vi "Real time state machine - Saccade suppression.vi"() -> ()   [LabVIEW 2013]
uses:
  <vilib>/Platform/TimedLoop/XDataNode/timing_clust.ctl
  <vilib>/Platform/TimedLoop/XDataNode/nitl_modes.ctl
  <vilib>/Platform/TimedLoop/XDataNode/wakeup.ctl
  <vilib>/DAQmx/write.llb/DAQmx Write (Digital 1D Bool NChan 1Samp 1Line).vi
  <vilib>/DAQmx/read.llb/DAQmx Read (Analog 1D DBL NChan 1Samp).vi
  <vilib>/platform/TimedLoop/XDataNode/XDataNode.xnode
  <vilib>/Platform/TimedLoop/XDataNode/XDNodeRunTimeDep.lvlib
panel:
  out "Min":dbl
  out "Sec":dbl=47.16078567504883
  in  "Display length (S)":sgl=10.0
  out "shaft encoder":waveform(sgl)(graph)={"t0"=timestamp(3524542772.3366966 s since 1904-01-01), "dt"=0.02, "Y"=array[500 elements]}
  out "Current state":T1(ring)=enum."VS"
  out "# of rewards":i32
  in  "Automatic reward":bool=TRUE
  out "Lick reward":bool
  out "RT FIFO (DISP)":u32(slide) scale=0.0..50.0
  out "RT FIFO (Log)":u32(slide) scale=0.0..50.0
  out "Digital Waveform Graph":digitalwaveform(graph)={"t0"=timestamp(3524542772.3366966 s since 1904-01-01), "dt"=0.0004, "Y"={"transitions"=[], "data"=array25000x3[75000 elements]}, "error"={"status"=FALSE, "code"=37421928, "source"=""}}
  out "Trial # (State machine)":u32=1
  out "Actual cycle period (uS)":i64=94
  in  "State machine cycle (uS)":i64=200
  in  "Save file to":string="C:\\ni-rt\\LabVIEW Data\\"
  in  "RT FIFO size":u32=50
  in  "VS filter period (uS)":i32=500
  out "Start one trial":bool
  out "Trial Done":bool
  out "error out":errorcluster
  out "Busy":bool
  out "Trial #":i32=1
  out "Save data":bool
  out "LED?":bool
  out "Pulse amp 0":sgl
  out "Pulse amp 1":sgl
  out "Pulse delay":sgl
  out "Pulse width":sgl
  out "Pulse period (ms)":sgl
  out "Pulse #":sgl
  out "Reward period (uS)":u32
  out "Reward start delay (uS)":u32
  out "Water duration (uS)":u32=30000
  out "Water refractory period (uS)":u32=500000
  out "Shock duration (uS)":u32=10000
  out "Shock refractory period (uS)":u32=1000000
  out "Trial timeout (uS)":u32=3000000
  out "Lick threshold (V)":fxp<+,32,16>=1.600006103515625
  out "Track eye":bool=TRUE
  out "Allow shock":bool
  out "Allow timeout":bool
  out "Manually give water":bool
  out "Manually give shock":bool
  out "VS threshold (V)":fxp<+,32,16>=0.5
  out "VS type":string="continuous_flash"
  out "File name":string="Test"
  out "Behavior type":string="fullfield"
  in  "Stop state":bool
  in  "Remote port":u16=9090
  in  "Remote IP_Main":string="192.168.137.10"
  in  "Local port":u16=9091
  in  "Local IP_This computer":string="192.168.137.2"
  out "ABORT":bool
  out "Initial data received":bool
  # "VS"
  # "Behavior"
  # "Trial #"
  # "Received parameters"
  # "Time to wait for reward window"
  # "Elapsed time"
  # "Min"
  # "Sec"
  # "Controls"
  # "Network"
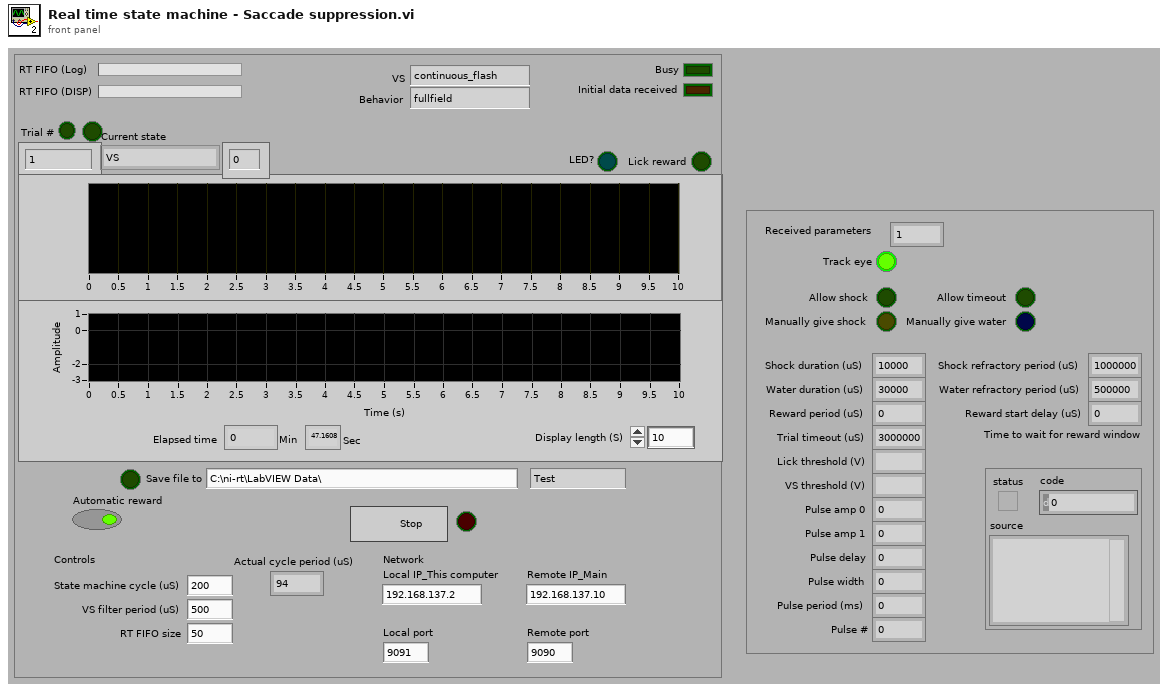
[diagram p1: front panel]
types:
  T1 = enum16{"Idle", "Before VS", "VS", "VS2", "After VS", "Wait for lever press", "Cycle End", "Reward", "Reward Refractory", "Punish", "Punish Refractory", "Exit", "Timeout", "Lick reward"}
  T2 = enum16{"open", "replace", "create", "open or create", "replace or create", "replace or create with confirmation"}
  T3 = typedef "XDNodeRunTimeDep.lvlib/timing_clust.ctl" = cluster{"Expected End [f-1]":u64, "Actual End [f-1]":u64, "Finished Late? [f-1]":bool, "Expected End [i-1]":u64, "Actual End [i-1]":u64, "Finished Late? [i-1]":bool, "Expected Start [i]":u64, "Actual Start [i]":u64, "Expected Start [f]":u64, "Actual Start [f]":u64, "Source Name":string, "Structure Name":string, "Period":i64, "Deadline":i64, "Offset":i64, "Start":i64, "Priority":i32, "Timeout":i32, "Mode":T4, "Wakeup Reason":T5, "Error":errorcluster, "Source Type":string, "Secondary Source Type":string, "Global End Time":u64, "Global Start Time":u64, "Frame Duration":u64, "Iteration Duration":u64, "Assigned CPU":i32, "I/O Scan Engine Mode":u32}
  T4 = typedef "XDNodeRunTimeDep.lvlib/nitl_modes.ctl" = enum32{"No Change", "Process missed periods, maintain original phase", "Discard missed periods, maintain original phase", "Process missed periods, ignore original phase", "Discard missed periods, ignore original phase"}
  T5 = typedef "XDNodeRunTimeDep.lvlib/wakeup.ctl" = enum32{"Normal", "Aborted", "Asynchronous wakeup", "Timing source error", "Timed loop error", "Timeout"}
  T6 = enum16{"big-endian, network order", "native, host order", "little-endian"}
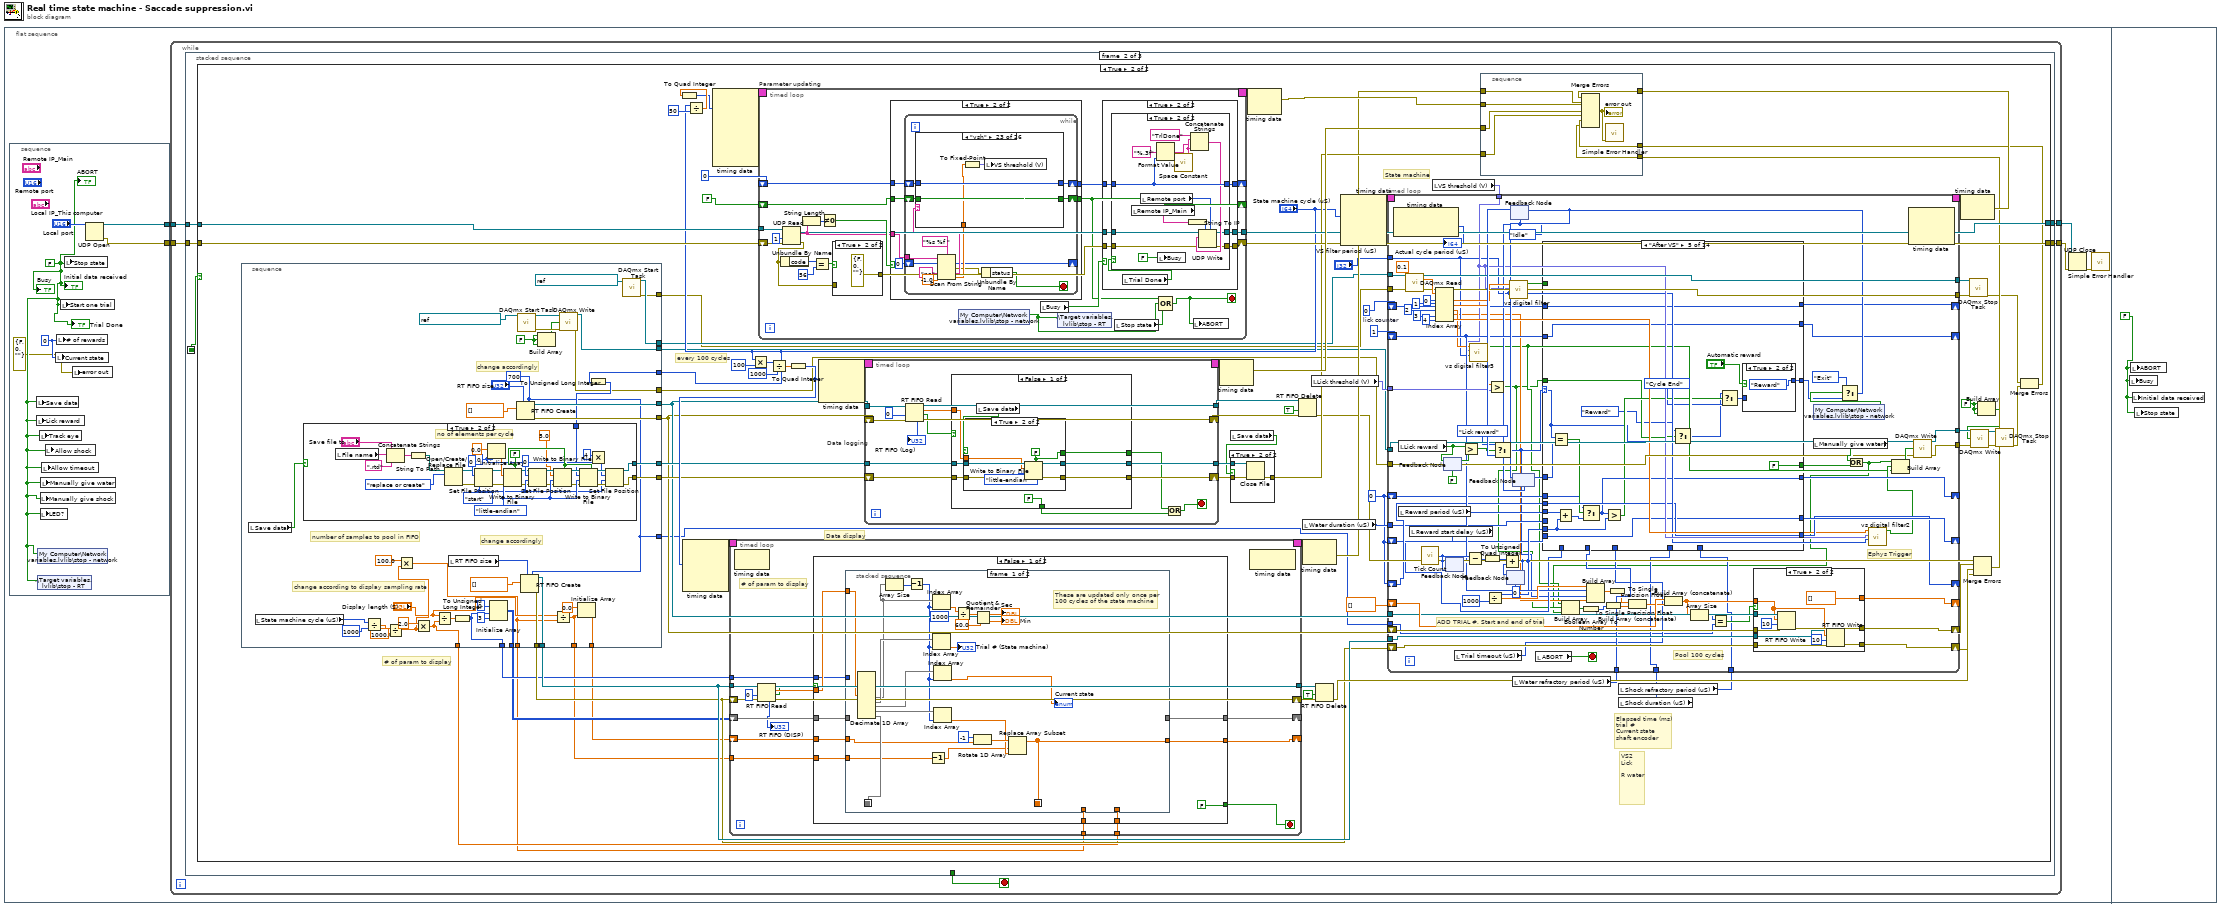
[diagram p0: block diagram]
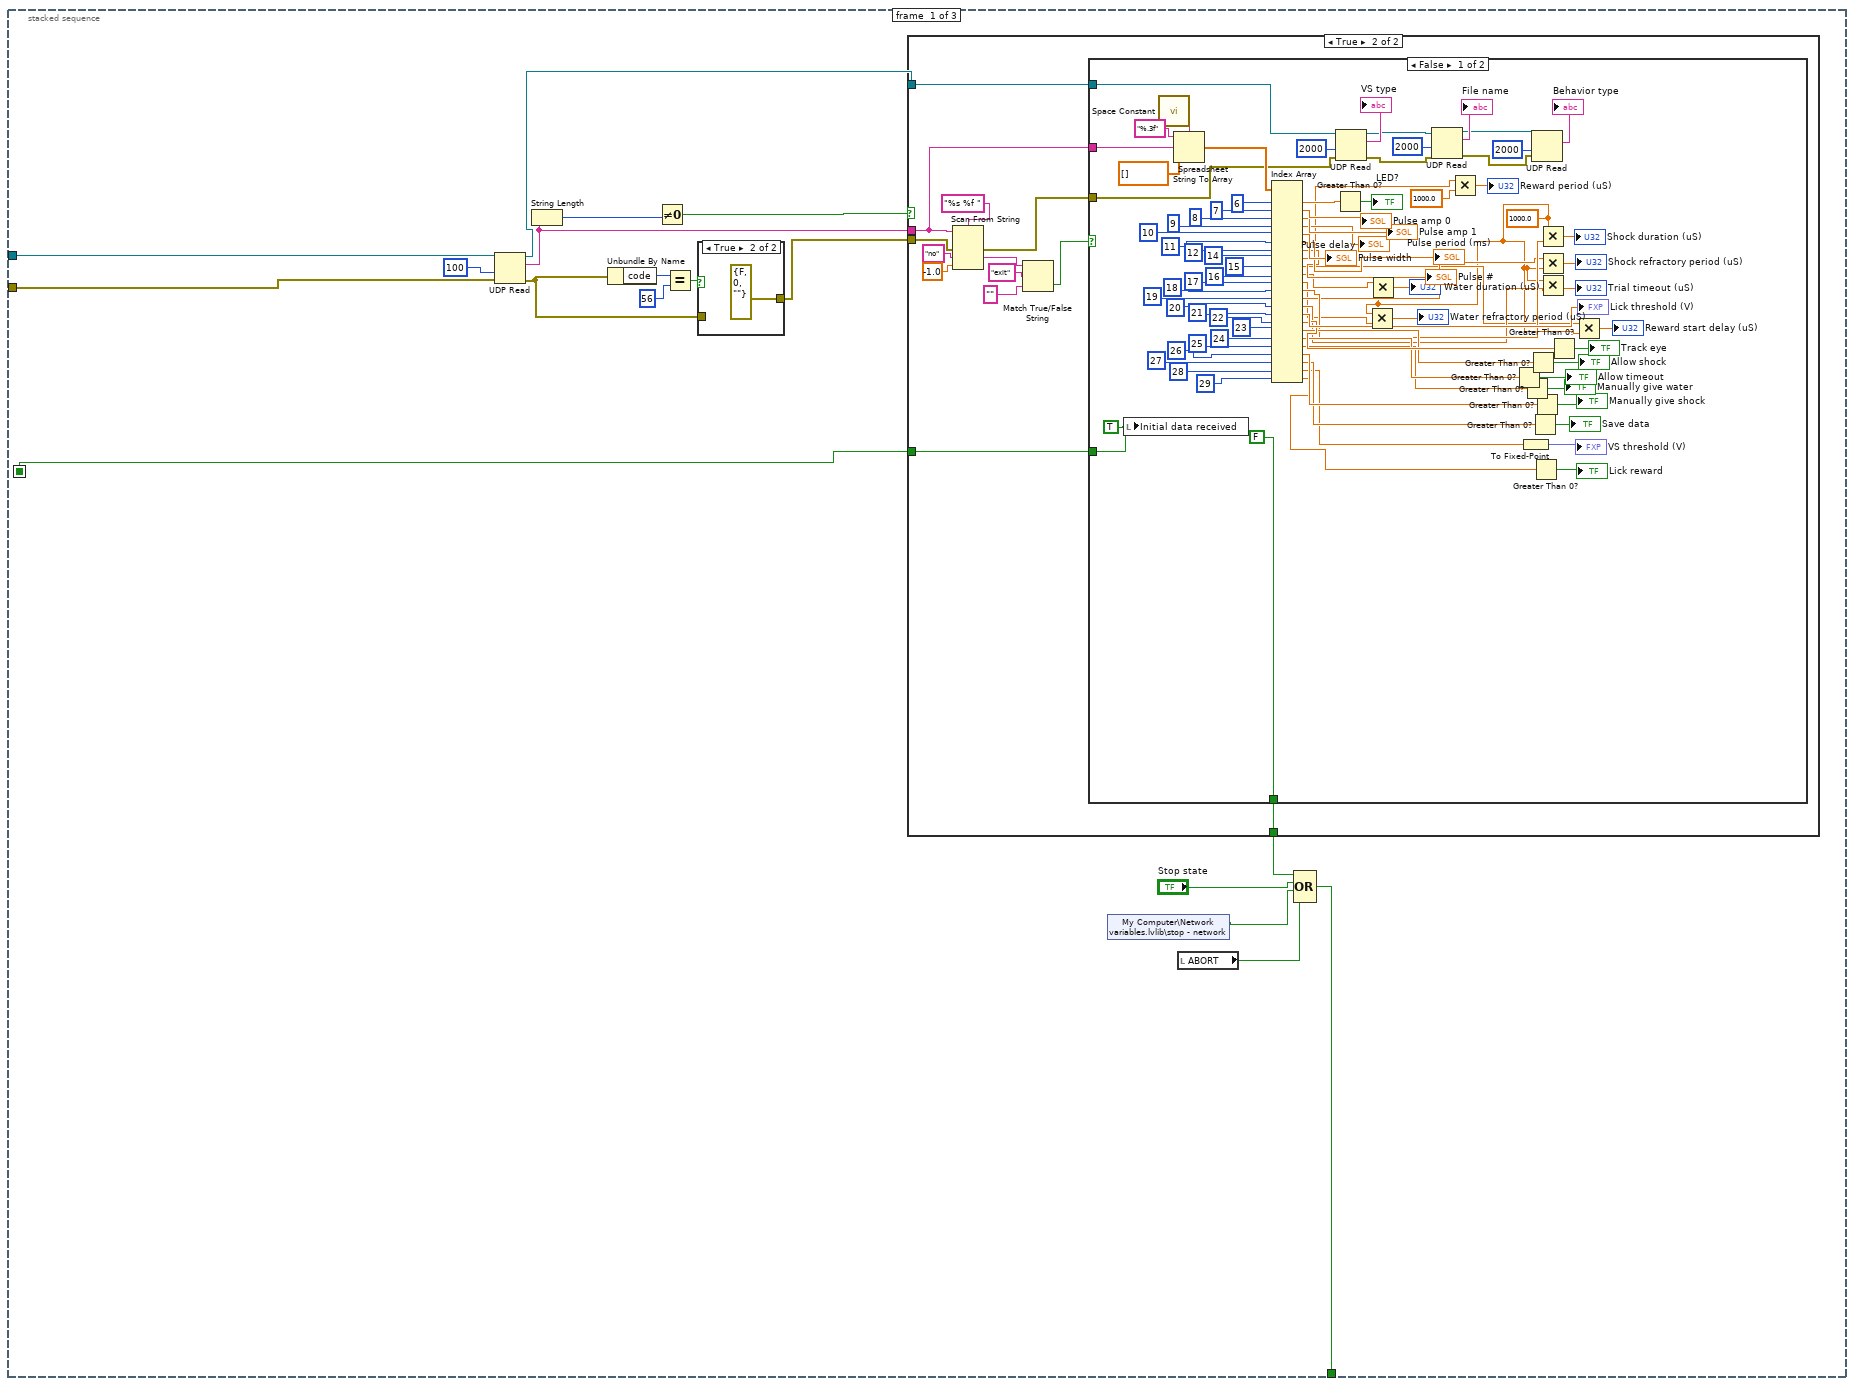
[diagram p2: hidden frame]
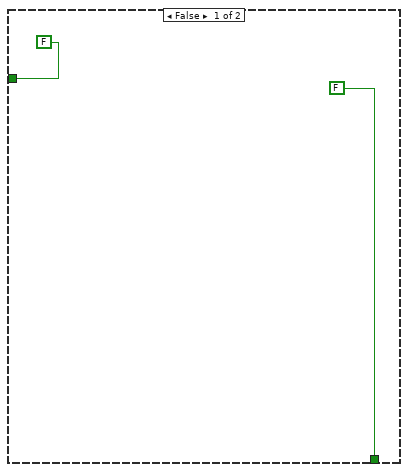
[diagram p3: hidden frame]
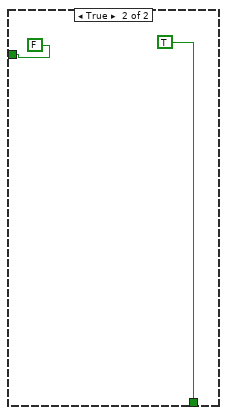
[diagram p4: hidden frame]
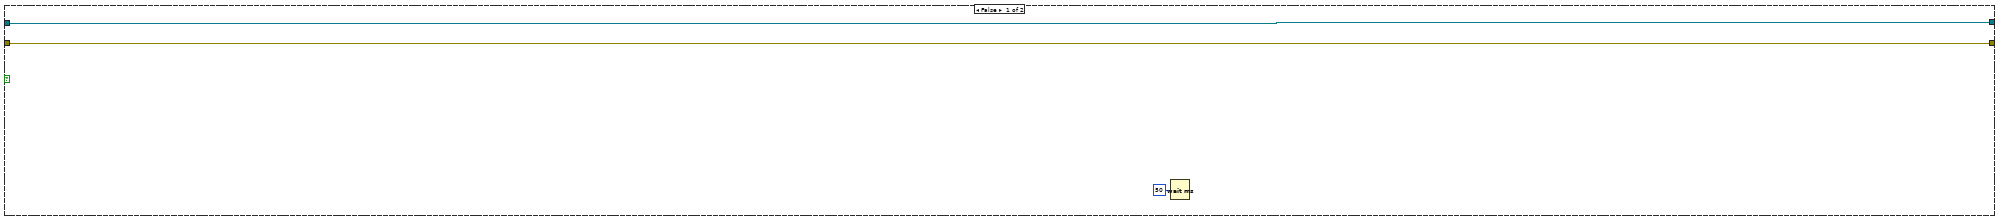
[diagram p6: hidden frame]
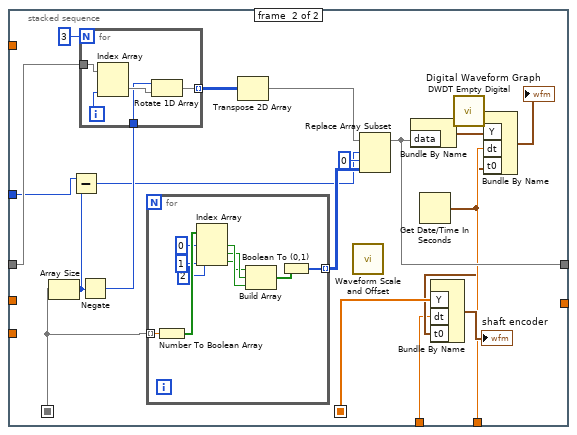
[diagram p9: hidden frame]
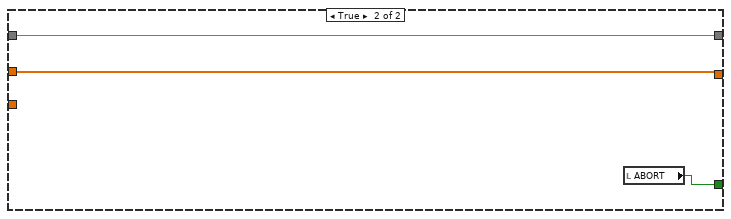
[diagram p10: hidden frame]
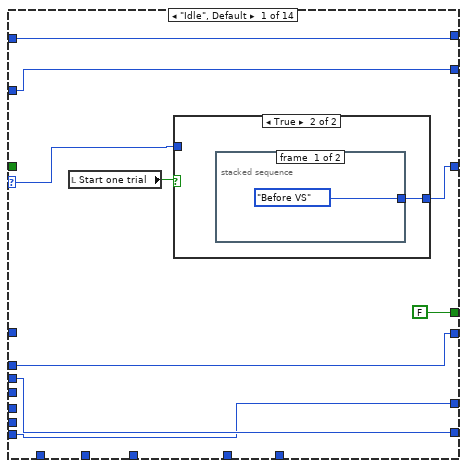
[diagram p11: hidden frame]
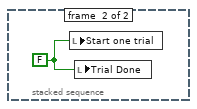
[diagram p13: hidden frame]
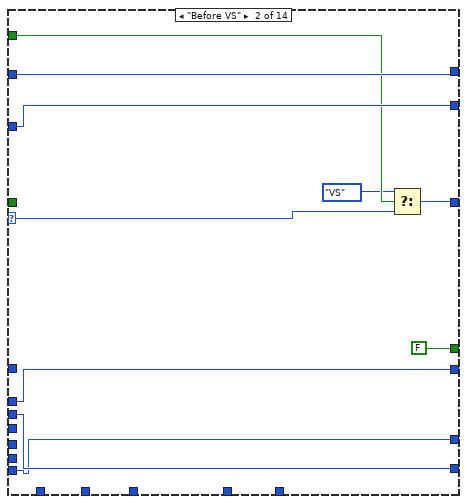
[diagram p14: hidden frame]
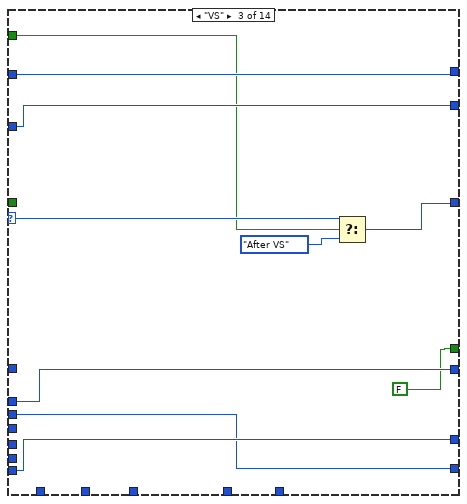
[diagram p15: hidden frame]
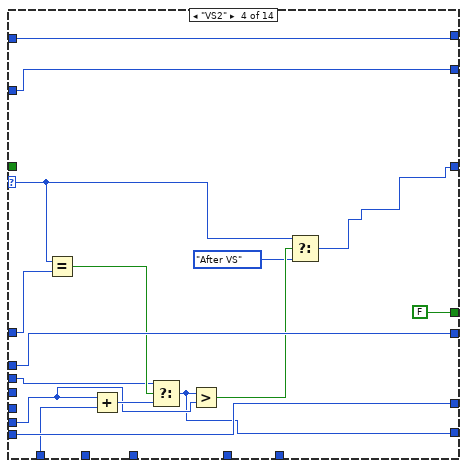
[diagram p16: hidden frame]
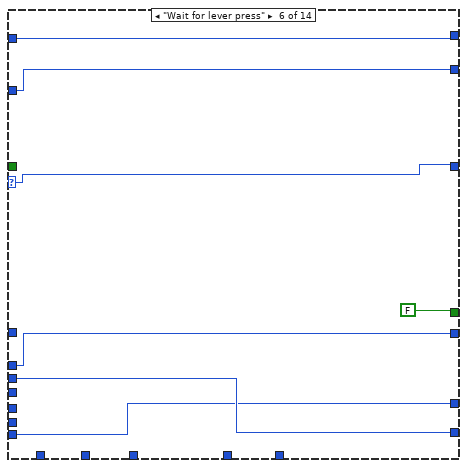
[diagram p18: hidden frame]
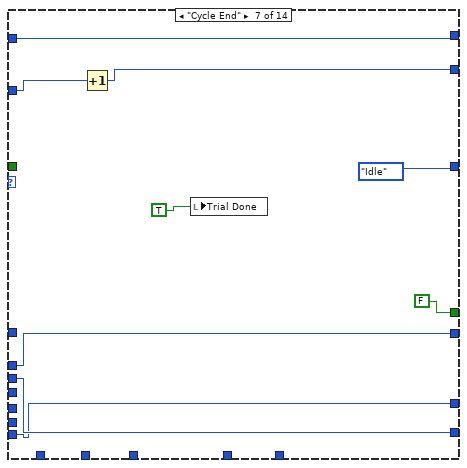
[diagram p19: hidden frame]
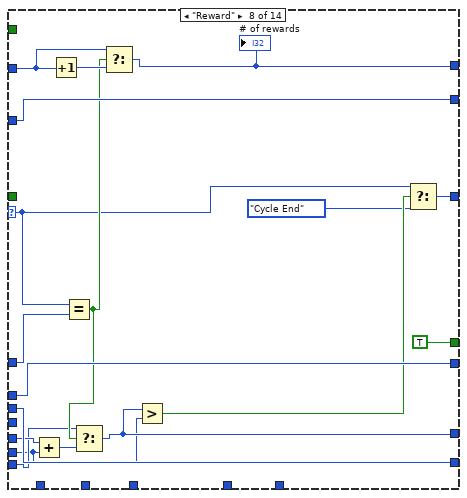
[diagram p20: hidden frame]
diagram:
  n1 = flat-sequence {
    frame #0 {
      n2 = stacked-sequence {
        tunnel: [w945] -> w5
        tunnel: [w944] -> w4
        frame #0 {
          w943 = 0
          w942 = FALSE
          n3 = local write "Save data"(w942) -> ()
          n4 = local write "Lick reward"(w942) -> ()
          n5 = shared-variable "My Computer\\Network variables.lvlib\\stop - network"(w942) -> ()  [unwired: 1 in, 1 out]
          n6 = shared-variable ".\\Target variables.lvlib\\stop - RT"(w942) -> ()  [unwired: 1 in, 1 out]
          n7 = local write "Track eye"(w942) -> ()
          n8 = local write "Manually give shock"(w942) -> ()
          n9 = local write "LED?"(w942) -> ()
          n10 = local write "Manually give water"(w942) -> ()
          n11 = local write "Allow timeout"(w942) -> ()
          n12 = local write "Allow shock"(w942) -> ()
          n13 = local write "Current state"(w943) -> ()
          n14 = local write "# of rewards"(w943) -> ()
          n15 = local write "Start one trial"(w942) -> ()
          n16 = local write "Stop state"(w942) -> ()
          n17 = local write "error out"(errorcluster {"status"=FALSE, "code"=0, "source"=""} ("error out")) -> ()
          n18 = UDP Open(11:"Local port") -> (port=w945:refnum<k16>, 0:w944:errorcluster)  [unwired: 4 in, 1 out]
          "ABORT" <- w942
          "Initial data received" <- w942
          "Busy" <- w942
          "Trial Done" <- w942
        }
      }
      n19 = while {
        tunnel: w5 -> [w10]
        tunnel: w4 -> [w9]
        tunnel: [w8] -> w3
        tunnel: [w7] -> w2
        stop <- w6 stop-if-true
        n20 = stacked-sequence {
          seq-local: [w16 _ _] -> [_ w135 _]
          tunnel: w10 -> [w27 w132 _]
          tunnel: w9 -> [w26 w133 _]
          tunnel: [w15 _ _] -> w6
          tunnel: [_ w134 _] -> w8
          tunnel: [_ w131 _] -> w7
          frame #0 {
            n21 = UDP Read(connection ID=w27, timeout ms (25000)=100, 8:w26) -> (data out=w18:string, error out=w22:errorcluster, 3:w17:refnum<k16>)  [unwired: 1 in, 2 out]
            n22 = String Length(string=w18) -> (length=w21:i32)
            n23 = Unbundle By Name(w22) -> ("code"=w25:i32)
            n24 = Not Equal To 0?(x=w21) -> (x != 0?=w20:bool)
            n25 = Equal?(x=w25, y=56) -> (x = y?=w23:bool)
            n26 = case shown="True" w23 {
              tunnel: w22 -> [w129 _]
              tunnel: [w129 errorcluster {"status"=FALSE, "code"=0, "source"=""} ("error out")] -> w19
              frame False {
              }
              frame True {
              }
            }
            n27 = case shown="True" w20 {
              tunnel: w19 -> [_ w41]
              tunnel: w18 -> [_ w35]
              tunnel: w17 -> [_ w33]
              tunnel: [FALSE w32] -> w14
              tunnel: [FALSE w31] -> w16
              frame False {
              }
              frame True {
                n28 = Scan From String(format string="%s %f ", input string=w35, error in=w41, default 1="no" ("default value 1"), default 2=sgl -1.0 ("default value 1")) -> (error out=w34:errorcluster, output 1=w39:string)  [unwired: 2 in, 2 out]
                n29 = Match True/False String(2:"" ("false string"), 3:"exit" ("true string"), 4:w39) -> (0:w36:bool)  [unwired: 1 out]
                n30 = case shown="False" w36 {
                  tunnel: w35 -> [w123 _]
                  tunnel: w34 -> [w81 _]
                  tunnel: w33 -> [w80 _]
                  tunnel: [FALSE TRUE] -> w32
                  tunnel: [w68 FALSE] -> w31
                  frame False {
                    w49 = sgl 1000.0
                    w68 = TRUE
                    n31 = local write "Initial data received"(w68) -> ()
                    n32 = call <vilib>:"Space Constant.vi"() -> ("String"=w125:string)
                    n33 = Spreadsheet String To Array(delimiter (Tab)=w125, format string="%.3f", spreadsheet string=w123, array type (2D Dbl)=sgl[] []) -> (array=w122:sgl[])
                    n34 = Index Array(array=w122, index #1=6 ("index"), index #2=7 ("index"), index #3=8 ("index"), index #4=9 ("index"), index #5=10 ("index"), index #6=11 ("index"), index #7=12 ("index"), index #8=14 ("index"), index #9=15 ("index"), index #10=16 ("index"), index #11=17 ("index"), index #12=18 ("index"), index #13=19 ("index"), index #14=20 ("index"), index #15=21 ("index"), index #16=22 ("index"), index #17=23 ("index"), index #18=24 ("index"), index #19=25 ("index"), index #20=26 ("index"), index #21=27 ("index"), index #22=28 ("index"), index #23=29 ("index")) -> (element #1=w120:sgl, element #2=→"Pulse amp 0":sgl, element #3=→"Pulse amp 1":sgl, element #4=→"Pulse delay":sgl, element #5=→"Pulse width":sgl, element #6=→"Pulse period (ms)":sgl, element #7=→"Pulse #":sgl, element #8=w64:sgl, element #9=w55:sgl, element #10=w53:sgl, element #11=w51:sgl, element #12=w61:sgl, element #13=w60:sgl, element #14=w57:sgl, element #15=→"Lick threshold (V)":sgl, element #16=w94:sgl, element #17=w91:sgl, element #18=w89:sgl, element #19=w86:sgl, element #20=w84:sgl, element #21=w46:sgl, element #22=w45:sgl, element #23=w44:sgl)
                    n35 = Greater Than 0?(x=w120) -> (x > 0?=→"LED?":bool)
                    n36 = UDP Read(connection ID=w80, timeout ms (25000)=2000, 8:w81) -> (data out=→"VS type":string, error out=w76:errorcluster, 3:w74:refnum<k16>)  [unwired: 1 in, 2 out]
                    n37 = Multiply(x=w49, y=w51) -> (x*y=→"Water refractory period (uS)":sgl)
                    n38 = Multiply(x=w53, y=w49) -> (x*y=→"Water duration (uS)":sgl)
                    n39 = UDP Read(connection ID=w74, timeout ms (25000)=2000, 8:w76) -> (data out=→"File name":string, error out=w72:errorcluster, 3:w71:refnum<k16>)  [unwired: 1 in, 2 out]
                    n40 = Multiply(x=w64, y=sgl 1000.0) -> (x*y=→"Reward period (uS)":sgl)
                    n41 = Greater Than 0?(x=w89) -> (x > 0?=→"Allow timeout":bool)
                    n42 = To Fixed-Point(number=w45) -> (fixed-point=→"VS threshold (V)":fxp<+/-,32,16>)  [unwired: 1 in]
                    n43 = Greater Than 0?(x=w86) -> (x > 0?=→"Manually give water":bool)
                    n44 = Greater Than 0?(x=w91) -> (x > 0?=→"Allow shock":bool)
                    n45 = Greater Than 0?(x=w46) -> (x > 0?=→"Save data":bool)
                    n46 = Greater Than 0?(x=w44) -> (x > 0?=→"Lick reward":bool)
                    n47 = UDP Read(connection ID=w71, timeout ms (25000)=2000, 8:w72) -> (data out=→"Behavior type":string)  [unwired: 1 in, 4 out]
                    n48 = Greater Than 0?(x=w84) -> (x > 0?=→"Manually give shock":bool)
                    n49 = Multiply(x=w49, y=w61) -> (x*y=→"Shock duration (uS)":sgl)
                    n50 = Multiply(x=w60, y=w49) -> (x*y=→"Shock refractory period (uS)":sgl)
                    n51 = Multiply(x=w49, y=w57) -> (x*y=→"Trial timeout (uS)":sgl)
                    n52 = Greater Than 0?(x=w94) -> (x > 0?=→"Track eye":bool)
                    n53 = Multiply(x=w55, y=w49) -> (x*y=→"Reward start delay (uS)":sgl)
                  }
                  frame True {
                  }
                }
              }
            }
            n54 = shared-variable "My Computer\\Network variables.lvlib\\stop - network"() -> (w11:bool)  [unwired: 1 in, 1 out]
            n55 = local read "ABORT"() -> (w12:bool)
            n56 = Compound Arithmetic op=OR(w14, "Stop state", w11, w12) -> (w15:bool)
          }
          frame #1 {
            n57 = case shown="True" w135 {
              tunnel: w133 -> [w138 w211]
              tunnel: [w138 w203] -> w134
              tunnel: w132 -> [w137 w210]
              tunnel: [w137 w202] -> w131
              frame False {
                n58 = Wait (ms)(milliseconds to wait=u32 50) -> ()  [unwired: 1 out]
              }
              frame True {
                w155 = FALSE
                w191 = 0  # lick counter
                w147 = 0
                # "every 100 cycles"
                # "VS2\nLick\n\nR water"
                # "# of param to display"
                # "Data display"
                # "Elapsed time (ms)\ntrial #\nCurrent state\nshaft encoder"
                # "State machine"
                n59 = stacked-sequence {
                  tunnel: [w264] -> w176
                  tunnel: [w263] -> w175
                  tunnel: [w260] -> w174
                  tunnel: [w259] -> w173
                  tunnel: [w245] -> w156
                  tunnel: [w240] -> w172
                  tunnel: [w251] -> w171
                  tunnel: "State machine cycle (uS)" -> [w244]
                  tunnel: [w248] -> w169
                  tunnel: [w247] -> w168
                  tunnel: [w242] -> w146
                  tunnel: [w239] -> w145
                  tunnel: [w235] -> w144
                  tunnel: [w234] -> w143
                  tunnel: [w232] -> w142
                  tunnel: [w231] -> w141
                  tunnel: [w225] -> w140
                  tunnel: [w224] -> w139
                  frame #0 {
                    w226 = FALSE
                    w242 = u32 700 ("elements in array (1)")
                    # "number of samples to pool in FIFO"
                    # "change according to display sampling rate"
                    # "change accordingly"
                    # "change accordingly"
                    n60 = local read "Save data"() -> (w265:bool)
                    n61 = local read "State machine cycle (uS)"() -> (w252:i64)
                    n62 = Divide(x=w252, y=u32 1000) -> (x/y=w254:dbl)
                    n63 = Divide(x=w254, y=1000.0) -> (x/y=w237:dbl)
                    n64 = Multiply(x=100.0, y=w237) -> (x*y=w235:dbl)
                    n65 = Multiply(x=2.0, y=w237) -> (x*y=w245:dbl)
                    n66 = Divide(x="Display length (S)", y=w245) -> (x/y=w257:dbl)
                    n67 = local read "RT FIFO size"() -> (w262:u32)
                    n68 = To Unsigned Long Integer(number=w257) -> (unsigned 32bit integer=w240:u32)
                    n69 = Initialize Array(u8 0 ("element"), w240, 3 ("dimension size")) -> (w251:u8[][])
                    n70 = RT FIFO Create(1:sgl[] [], 4:"RT FIFO size", 6:w242) -> (8:w248:refnum<k33>, 11:w247:errorcluster)  [unwired: 5 in, 1 out]
                    n71 = call <vilib>:"DAQmx Start Task.vi"("task/channels in"=refnum<k21> "Digital_write_saccade" ("DAQmx Task Name")) -> ("task out"=w229:refnum<k21>, "error out"=w228:errorcluster)  [unwired: 13 in]
                    n72 = RT FIFO Create(1:sgl[] [], 4:w262, 6:w242) -> (8:w260:refnum<k33>, 11:w259:errorcluster)  [unwired: 5 in, 1 out]
                    n73 = Build Array(w226, w226, w226) -> (w227:bool[])
                    n74 = Divide(x="Display length (S)", y=w235) -> (x/y=w234:dbl)
                    n75 = call-poly <vilib>:"DAQmx Write.vi"("task/channels in"=w229, "data"=w227, "error in"=w228) -> ("task out"=w225:refnum<k21>, "error out"=w224:errorcluster)  [unwired: 10 in, 1 out]
                    n76 = Initialize Array(sgl 0.0 ("element"), w234) -> (w239:sgl[])
                    n77 = To Unsigned Long Integer(number=w244) -> (unsigned 32bit integer=w243:u32)
                    n78 = case shown="True" w265 {
                      tunnel: [_ w269] -> w264
                      tunnel: [_ w268] -> w263
                      tunnel: w243 -> [_ w267]
                      frame False {
                      }
                      frame True {
                        w290 = FALSE
                        w283 = 10 ("dimension size")
                        w291 = T6."little-endian" ("byte order (0:big-endian, network order)")
                        w282 = enum16{"start", "end", "current"}."start" ("from (0:start)")
                        # "no of elements per cycle"
                        n79 = local read "File name"() -> (w293:string)
                        n80 = Concatenate Strings("Save file to", w293, ".rtd" ("string")) -> (w296:string)
                        n81 = String To Path(string=w296) -> (path=w297:path)
                        n82 = Open/Create/Replace File(file path (use dialog)=w297, operation (0:open)=T2."replace or create") -> (refnum out=w270:refnum<file>, error out=w271:errorcluster)  [unwired: 4 in, 1 out]
                        n83 = Set File Position(offset (in bytes) (0)=i64 0, refnum=w270, from (0:start)=w282, error in=w271) -> (refnum out=w273:refnum<file>, error out=w274:errorcluster)
                        n84 = Initialize Array(sgl 0.0 ("element"), w283) -> (w276:sgl[])
                        n85 = Write to Binary File(file (use dialog)=w273, data=w276, error in=w274, 5:w290, 9:w291) -> (refnum out=w278:refnum<file>, error out=w277:errorcluster)  [unwired: 1 in, 1 out]
                        n86 = Set File Position(offset (in bytes) (0)=i64 0, refnum=w278, from (0:start)=w282, error in=w277) -> (refnum out=w280:refnum<file>, error out=w281:errorcluster)
                        n87 = Write to Binary File(file (use dialog)=w280, data=sgl 5.0, error in=w281, 5:w290, 9:w291) -> (refnum out=w288:refnum<file>, error out=w286:errorcluster)  [unwired: 1 in, 1 out]
                        n88 = Write to Binary File(file (use dialog)=w288, data=w267, error in=w286, 5:w290, 9:w291) -> (refnum out=w289:refnum<file>, error out=w287:errorcluster)  [unwired: 1 in, 1 out]
                        n89 = Multiply(x=4, y=w283) -> (x*y=w285:i32)
                        n90 = Set File Position(offset (in bytes) (0)=w285, refnum=w289, from (0:start)=w282, error in=w287) -> (refnum out=w268:refnum<file>, error out=w269:errorcluster)
                      }
                    }
                    n91 = call <vilib>:"DAQmx Start Task.vi"("task/channels in"=refnum<k21> "Analog_read_saccade" ("DAQmx Task Name")) -> ("task out"=w232:refnum<k21>, "error out"=w231:errorcluster)  [unwired: 13 in]
                  }
                }
                n92 = Divide(x="State machine cycle (uS)", y=i64 50) -> (x/y=w181:dbl)
                n93 = To Quad Integer(1:w181) -> (0:w180:i64)
                n94 = node-c288 ("Input Node")(w180) -> (w219:T3)  [unwired: 6 in]
                n95 = Multiply(x="State machine cycle (uS)", y=u32 100) -> (x*y=w184:i64)
                n96 = timed-loop "Parameter updating" {
                  timing: w219 -> [_]
                  timing-out: [_] -> w218
                  tunnel: w210 -> [w778]
                  shift-right: [w763] -> w203
                  shift-left: w211 -> [w779]
                  shift-right: [w766] -> _
                  shift-left: 0 -> [w769]
                  tunnel: [w762] -> w202
                  shift-right: [w760] -> _
                  shift-left: FALSE -> [w770]
                  stop <- w761 stop-if-true
                  n97 = UDP Read(connection ID=w778, timeout ms (25000)=1, 8:w779) -> (data out=w771:string, error out=w774:errorcluster, 3:w764:refnum<k16>)  [unwired: 1 in, 2 out]
                  n98 = Unbundle By Name(w774) -> ("code"=w777:i32)
                  n99 = String Length(string=w771) -> (length=w773:i32)
                  n100 = Equal?(x=w777, y=56) -> (x = y?=w775:bool)
                  n101 = Not Equal To 0?(x=w773) -> (x != 0?=w772:bool)
                  n102 = case shown="True" w775 {
                    tunnel: w774 -> [w931 _]
                    tunnel: [w931 errorcluster {"status"=FALSE, "code"=0, "source"=""} ("error out")] -> w765
                    frame False {
                    }
                    frame True {
                    }
                  }
                  n103 = case shown="True" w772 {
                    tunnel: w771 -> [_ w814]
                    tunnel: w770 -> [w807 w813]
                    tunnel: w769 -> [w808 w812]
                    tunnel: [w808 w811] -> w767
                    tunnel: [w807 w810] -> w760
                    frame False {
                    }
                    frame True {
                      n104 = while {
                        tunnel: w814 -> [w826]
                        shift-right: [w822] -> w810
                        shift-left: w813 -> [w823]
                        shift-right: [w821] -> w811
                        shift-left: w812 -> [w820]
                        shift-right: [w816] -> _
                        shift-left: u32 0 -> [w817]
                        stop <- w818 stop-if-true
                        n105 = Scan From String(format string="%s %f ", input string=w826, initial scan location=w817, default 1="no" ("default value 1"), default 2=-1.0 ("default value 2")) -> (offset past scan=w816:u32, error out=w819:errorcluster, output 1=w825:string, output 2=w824:dbl)  [unwired: 1 in, 1 out]
                        n106 = case shown="\"vsh\"" w825 {
                          tunnel: w824 -> [_ w833 w837 w840 w843 w846 w849 w852 w854 w858 w863 w869 w874 w879 w884 w890 w893 w897 w902 w905 w909 w913 w916 w920 _ _]
                          tunnel: w823 -> [w830 w831 w835 w838 w841 w844 w847 w850 w856 w861 w866 w871 w876 w881 w886 w888 w891 w895 w899 w903 w907 w911 w917 w921 w924 w929]
                          tunnel: [w830 w831 w835 w838 w841 w844 w847 w850 w856 w861 w866 w871 w876 w881 w886 w888 w891 w895 w899 w903 w907 w911 w917 w921 w924 w928] -> w822
                          tunnel: [w829 w832 w836 w839 w842 w845 w848 w851 w857 w862 w867 w872 w877 w882 w887 w889 w892 w896 w900 w904 w908 w912 w918 w922 w925 w927] -> w821
                          tunnel: w820 -> [w829 w832 w836 w839 w842 w845 w848 w851 w857 w862 w867 w872 w877 w882 w887 w889 w892 w896 w900 w904 w908 w912 w918 w922 w926 w927]
                          frame "no", Default {
                          }
                          frame "led" {
                            n107 = Greater Than 0?(x=w833) -> (x > 0?=w834:bool)
                            n108 = local write "LED?"(w834) -> ()
                          }
                          frame "pai" {
                            n109 = local write "Pulse amp 0"(w837) -> ()
                          }
                          frame "paf" {
                            n110 = local write "Pulse amp 1"(w840) -> ()
                          }
                          frame "pdl" {
                            n111 = local write "Pulse delay"(w843) -> ()
                          }
                          frame "pwd" {
                            n112 = local write "Pulse width"(w846) -> ()
                          }
                          frame "ppr" {
                            n113 = local write "Pulse period (ms)"(w849) -> ()
                          }
                          frame "pnm" {
                            n114 = local write "Pulse #"(w852) -> ()
                          }
                          frame "rwp" {
                            n115 = Multiply(x=1000.0, y=w854) -> (x*y=w853:dbl)
                            n116 = local write "Reward period (uS)"(w853) -> ()
                          }
                          frame "rwd" {
                            n117 = Multiply(x=1000.0, y=w858) -> (x*y=w859:dbl)
                            n118 = local write "Reward start delay (uS)"(w859) -> ()
                          }
                          frame "wdr" {
                            n119 = Multiply(x=1000.0, y=w863) -> (x*y=w864:dbl)
                            n120 = local write "Water duration (uS)"(w864) -> ()
                          }
                          frame "wre" {
                            n121 = Multiply(x=1000.0, y=w869) -> (x*y=w868:dbl)
                            n122 = local write "Water refractory period (uS)"(w868) -> ()
                          }
                          frame "shd" {
                            n123 = Multiply(x=1000.0, y=w874) -> (x*y=w873:dbl)
                            n124 = local write "Shock duration (uS)"(w873) -> ()
                          }
                          frame "shr" {
                            n125 = Multiply(x=1000.0, y=w879) -> (x*y=w878:dbl)
                            n126 = local write "Shock refractory period (uS)"(w878) -> ()
                          }
                          frame "tto" {
                            n127 = Multiply(x=1000.0, y=w884) -> (x*y=w883:dbl)
                            n128 = local write "Trial timeout (uS)"(w883) -> ()
                          }
                          frame "lkt" {
                            n129 = local write "Lick threshold (V)"(w890) -> ()
                          }
                          frame "etk" {
                            n130 = Greater Than 0?(x=w893) -> (x > 0?=w894:bool)
                            n131 = local write "Track eye"(w894) -> ()
                          }
                          frame "ash" {
                            n132 = Greater Than 0?(x=w897) -> (x > 0?=w898:bool)
                            n133 = local write "Allow shock"(w898) -> ()
                          }
                          frame "ato" {
                            n134 = Greater Than 0?(x=w902) -> (x > 0?=w901:bool)
                            n135 = local write "Allow timeout"(w901) -> ()
                          }
                          frame "gwt" {
                            n136 = Greater Than 0?(x=w905) -> (x > 0?=w906:bool)
                            n137 = local write "Manually give water"(w906) -> ()
                          }
                          frame "gsh" {
                            n138 = Greater Than 0?(x=w909) -> (x > 0?=w910:bool)
                            n139 = local write "Manually give shock"(w910) -> ()
                          }
                          frame "sav" {
                            n140 = Greater Than 0?(x=w913) -> (x > 0?=w914:bool)
                            n141 = local write "Save data"(w914) -> ()
                          }
                          frame "vsh" {
                            n142 = To Fixed-Point(number=w916) -> (fixed-point=w915:fxp<+/-,32,16>)  [unwired: 1 in]
                            n143 = local write "VS threshold (V)"(w915) -> ()
                          }
                          frame "rew" {
                            n144 = Greater Than 0?(x=w920) -> (x > 0?=w919:bool)
                            n145 = local write "Lick reward"(w919) -> ()
                          }
                          frame "start" {
                            w923 = TRUE
                            n146 = Increment(x=w926) -> (x+1=w925:i32)
                            "Trial #" <- w925
                            n147 = local write "Busy"(w923) -> ()
                            "Start one trial" <- w923
                          }
                          frame "stop" {
                            n148 = Or(x=w929, y=TRUE) -> (x .or. y?=w928:bool)
                          }
                        }
                        n149 = Unbundle By Name(w819) -> ("status"=w818:bool)
                      }
                    }
                  }
                  n150 = shared-variable "My Computer\\Network variables.lvlib\\stop - network"() -> (w758:bool)  [unwired: 1 in, 1 out]
                  n151 = local read "Busy"() -> (w768:bool)
                  n152 = shared-variable ".\\Target variables.lvlib\\stop - RT"(w758) -> ()  [unwired: 1 in, 1 out]
                  n153 = case shown="True" w768 {
                    tunnel: w767 -> [w782 w788]
                    tunnel: [w782 w787] -> w766
                    tunnel: w765 -> [w780 w786]
                    tunnel: w764 -> [w781 w785]
                    tunnel: [w780 w784] -> w763
                    tunnel: [w781 w783] -> w762
                    frame False {
                    }
                    frame True {
                      n154 = local read "Trial Done"() -> (w789:bool)
                      n155 = case shown="True" w789 {
                        tunnel: [w792 w800] -> w787
                        tunnel: w788 -> [w792 w800]
                        tunnel: w786 -> [w791 w797]
                        tunnel: w785 -> [w790 w796]
                        tunnel: [w791 w794] -> w784
                        tunnel: [w790 w793] -> w783
                        frame False {
                        }
                        frame True {
                          n156 = local read "Remote IP_Main"() -> (w805:string)
                          n157 = local read "Remote port"() -> (w804:u16)
                          n158 = Format Value(format string="%.3f", value (0)=w800) -> (output string=w799:string)  [unwired: 1 in]
                          n159 = local write "Busy"(FALSE) -> ()
                          n160 = call <vilib>:"Space Constant.vi"() -> ("String"=w802:string)
                          n161 = String To IP(1:w805) -> (0:w806:u32)
                          n162 = Concatenate Strings("TrlDone" ("data in"), w802, w799, w802) -> (w798:string)
                          n163 = UDP Write(address=w806, port or service name=w804, connection ID=w796, data in=w798, 8:w797) -> (error out=w794:errorcluster, 3:w793:refnum<k16>)  [unwired: 1 in]
                        }
                      }
                    }
                  }
                  n164 = local read "Stop state"() -> (w759:bool)
                  n165 = Compound Arithmetic op=OR(w760, w758, w759) -> (w761:bool)
                  n166 = local write "ABORT"(w761) -> ()
                }
                n167 = Divide(x=w184, y=u32 1000) -> (x/y=w179:dbl)
                n168 = To Quad Integer(1:w179) -> (0:w178:i64)
                n169 = node-c288(w178) -> (w205:T3)  [unwired: 3 in]
                n170 = timed-loop {
                  timing: w205 -> [_]
                  timing-out: [_] -> w204
                  shift-right: [w311] -> w189
                  shift-left: w173 -> [w312]
                  tunnel: w174 -> [w314]
                  tunnel: [w313] -> w190
                  tunnel: w172 -> [w306]
                  shift-right: [w305] -> _
                  shift-left: w171 -> [w307]
                  tunnel: w156 -> [w304]
                  shift-right: [w300] -> _
                  shift-left: w145 -> [w301]
                  tunnel: w144 -> [w299]
                  tunnel: w143 -> [w298]
                  stop <- w302 stop-if-true
                  # "# of param to display"
                  n171 = node-c288() -> ()  [unwired: 1 in, 1 out]
                  n172 = RT FIFO Read(0:w314, 2:0 ("timeout in ms (0)"), 3:w312) -> (7:→"RT FIFO (DISP)":u32, 8:w313:refnum<k33>, 9:w309:sgl[], 10:w308:bool, 11:w311:errorcluster)  [unwired: 1 in]
                  n173 = case shown="False" w308 {
                    tunnel: w309 -> [w324 _]
                    tunnel: w307 -> [w323 w385]
                    tunnel: w306 -> [w322 _]
                    tunnel: [w321 w385] -> w305
                    tunnel: w304 -> [w320 _]
                    tunnel: [FALSE w384] -> w302
                    tunnel: w301 -> [w318 w383]
                    tunnel: [w317 w383] -> w300
                    tunnel: w299 -> [w316 _]
                    tunnel: w298 -> [w315 _]
                    frame False {
                      n174 = stacked-sequence {
                        seq-local: [w334 _] -> [_ w364]
                        seq-local: [w326 _] -> [_ w350]
                        tunnel: w324 -> [w347 _]
                        tunnel: w323 -> [_ w366]
                        tunnel: w322 -> [_ w359]
                        tunnel: [_ w356] -> w321
                        tunnel: w320 -> [_ w351]
                        tunnel: w318 -> [w331 _]
                        tunnel: [w326 _] -> w317
                        tunnel: w316 -> [_ w348]
                        tunnel: w315 -> [w325 _]
                        frame #0 {
                          # "These are updated only once per \n100 cycles of the state machine"
                          n175 = Decimate 1D Array(w347) -> (w336:sgl[], w337:sgl[], w338:sgl[], w333:sgl[], w334:sgl[])  [unwired: 5 out]
                          n176 = Array Size(array=w336) -> (size(s)=w346:i32)
                          n177 = Decrement(x=w346) -> (x-1=w332:i32)
                          n178 = Decrement(x=w325) -> (x-1=w327:dbl)
                          n179 = Index Array(array=w336, index=w332) -> (element=w345:sgl)
                          n180 = Index Array(array=w337, index=w332) -> (element=→"Trial # (State machine)":sgl)
                          n181 = Index Array(array=w338, index=w332) -> (element=→"Current state":sgl)
                          n182 = Index Array(array=w333, index=w332) -> (element=w329:sgl)
                          n183 = Divide(x=w345, y=u32 1000) -> (x/y=w343:sgl)
                          n184 = Rotate 1D Array(1:w331, 2:-1 ("n")) -> (0:w330:sgl[])
                          n185 = Quotient & Remainder(x=w343, y=60.0) -> (x-y*floor(x/y)=→"Sec":dbl, floor(x/y)=→"Min":dbl)
                          n186 = Replace Array Subset(array=w330, new element=w329, index=w327) -> (w326:sgl[])
                        }
                        frame #1 {
                          n187 = Array Size(array=w364) -> (size(s)=w358:i32)
                          n188 = Subtract(x=w359, y=w358) -> (x-y=w357:u32)
                          n189 = Negate(x=w358) -> (-x=w365:i32)
                          n190 = for {
                            N: 3 -> [_]
                            tunnel: w366 -> [w382]
                            tunnel: w365 -> [w379]
                            tunnel: [w378] -> w362 mode=indexing
                            i -> [w381]
                            n191 = Index Array(array=w382, index (col)=w381) -> (element=w380:u8[])  [unwired: 1 in]
                            n192 = Rotate 1D Array(1:w380, 2:w379) -> (0:w378:u8[])
                          }
                          n193 = for {
                            tunnel: w364 -> [w377] mode=indexing
                            tunnel: [w371] -> w363 mode=indexing
                            n194 = Number To Boolean Array(number=w377) -> (Boolean array=w376:bool[])
                            n195 = Index Array(array=w376, index #1=0 ("index"), index #2=1 ("index"), index #3=2 ("index")) -> (element #1=w370:bool, element #2=w369:bool, element #3=w368:bool)
                            n196 = Build Array(w368, w369, w370) -> (w372:bool[])
                            n197 = Boolean To (0,1)(Boolean=w372) -> (0, 1=w371:i16[])
                          }
                          n198 = Transpose 2D Array(2D array=w362) -> (transposed array=w361:u8[][])
                          n199 = call <vilib>:"Waveform Scale and Offset.vi"() -> ()  [unwired: 10 in, 2 out]
                          n200 = Replace Array Subset(array=w361, new element=w363, index (row)=w357, index (col)=0 ("disabled index (col)")) -> (w356:u8[][])
                          n201 = Bundle By Name("data"=w356) -> (w355:digitaldata)  [unwired: 1 in]
                          n202 = Get Date/Time In Seconds() -> (seconds since 1Jan1904=w349:timestamp)
                          n203 = Bundle By Name("Y"=w350, "dt"=w348, "t0"=w349) -> (→"shaft encoder":waveform(sgl))  [unwired: 1 in]
                          n204 = call <vilib>:"DWDT Empty Digital.vi"() -> ("digital waveform out"=w354:digitalwaveform)  [unwired: 5 in]
                          n205 = Bundle By Name(cluster=w354, "Y"=w355, "dt"=w351, "t0"=w349) -> (→"Digital Waveform Graph":digitalwaveform)
                        }
                      }
                    }
                    frame True {
                      n206 = local read "ABORT"() -> (w384:bool)
                    }
                  }
                  n207 = node-c288() -> ()  [unwired: 1 in, 1 out]
                }
                n208 = node-c288 ("Input Node")(w178) -> (w217:T3)  [unwired: 2 in]
                n209 = timed-loop "Data logging" {
                  timing: w217 -> [_]
                  timing-out: [_] -> w216
                  tunnel: [w727] -> w212
                  tunnel: w175 -> [w725]
                  tunnel: w169 -> [w722]
                  shift-right: [w721] -> w194
                  shift-left: w168 -> [w723]
                  tunnel: [w719] -> w192
                  shift-right: [w726] -> w213
                  shift-left: w176 -> [w724]
                  stop <- w715 stop-if-true
                  n210 = RT FIFO Read(0:w722, 2:0 ("timeout in ms (0)"), 3:w723) -> (7:→"RT FIFO (Log)":u32, 8:w719:refnum<k33>, 9:w717:sgl[], 10:w718:bool, 11:w721:errorcluster)  [unwired: 1 in]
                  n211 = case shown="False" w718 {
                    tunnel: [w735 w748] -> w727
                    tunnel: [w734 w749] -> w726
                    tunnel: w725 -> [w733 w748]
                    tunnel: w724 -> [w732 w749]
                    tunnel: w717 -> [w730 _]
                    tunnel: [FALSE w746] -> w713
                    tunnel: [w728 FALSE] -> w714
                    frame False {
                      n212 = local read "Save data"() -> (w731:bool)
                      n213 = case shown="True" w731 {
                        tunnel: [w738 w745] -> w735
                        tunnel: [w737 w744] -> w734
                        tunnel: w733 -> [w738 w743]
                        tunnel: w732 -> [w737 w742]
                        tunnel: w730 -> [_ w741]
                        tunnel: [w736 w739] -> w728
                        frame False {
                          n214 = local read "ABORT"() -> (w736:bool)
                        }
                        frame True {
                          w739 = FALSE
                          n215 = Write to Binary File(file (use dialog)=w743, data=w741, error in=w742, 5:w739, 9:T6."little-endian" ("byte order (0:big-endian, network order)")) -> (refnum out=w745:refnum<file>, error out=w744:errorcluster)  [unwired: 1 in, 1 out]
                        }
                      }
                    }
                    frame True {
                      n216 = local read "ABORT"() -> (w746:bool)
                    }
                  }
                  n217 = Or(x=w714, y=w713) -> (x .or. y?=w715:bool)
                }
                n218 = node-c288 ("Output Node")(w216) -> (w215:errorcluster)
                n219 = local read "Save data"() -> (w165:bool)
                n220 = case shown="True" w165 {
                  tunnel: w213 -> [w220 w223]
                  tunnel: w212 -> [_ w222]
                  tunnel: [w220 w221] -> w201
                  frame False {
                  }
                  frame True {
                    n221 = Close File(refnum=w222, error in=w223) -> (error out=w221:errorcluster)  [unwired: 1 out]
                  }
                }
                n222 = node-c288 ("Output Node")(w218) -> (w214:errorcluster)
                n223 = RT FIFO Delete(0:w192, 2:TRUE ("force destroy? (F)"), 3:w194) -> (11:w193:errorcluster)
                n224 = node-c288(w204) -> (w200:errorcluster)
                n225 = local read "Water duration (uS)"() -> (w151:u32)
                n226 = local read "Lick threshold (V)"() -> (w152:fxp<+,32,16>)
                n227 = RT FIFO Delete(0:w190, 2:TRUE ("force destroy? (F)"), 3:w189) -> (11:w188:errorcluster)
                n228 = node-c288("State machine cycle (uS)") -> (w207:T3)  [unwired: 3 in]
                n229 = local read "VS threshold (V)"() -> (w153:fxp<+,32,16>)
                n230 = local read "Water refractory period (uS)"() -> (w148:u32)
                n231 = local read "Shock refractory period (uS)"() -> (w150:u32)
                n232 = local read "Shock duration (uS)"() -> (w149:u32)
                n233 = timed-loop {
                  timing: w207 -> [_]
                  timing-out: [_] -> w206
                  shift-right: [w420] -> _
                  shift-left: w147 -> [w434]
                  shift-right: [w422] -> _
                  shift-left: 1 -> [w435]
                  shift-right: [w419] -> _
                  shift-left: w147 -> [w429]
                  tunnel: w169 -> [w466]
                  shift-right: [w465] -> w196
                  shift-left: w168 -> [w464]
                  shift-right: [w423] -> _
                  shift-left: w191 -> [w436]
                  tunnel: w174 -> [w461]
                  shift-right: [w459] -> w187
                  shift-left: w173 -> [w460]
                  shift-right: [w462] -> _
                  shift-left: sgl[] [] ("array type (2D Dbl)") -> [w467]
                  tunnel: w142 -> [w452]
                  tunnel: w141 -> [w451]
                  tunnel: [w446] -> w164
                  tunnel: [w445] -> w163
                  tunnel: w140 -> [w443]
                  tunnel: w139 -> [w442]
                  tunnel: [w441] -> w160
                  tunnel: [w440] -> w161
                  tunnel: "VS filter period (uS)" -> [w404]
                  tunnel: w153 -> [w405]
                  tunnel: w152 -> [w438]
                  tunnel: w151 -> [w431]
                  tunnel: w150 -> [w424]
                  tunnel: w149 -> [w425]
                  tunnel: w148 -> [w427]
                  shift-right: [w418] -> _
                  shift-left: w147 -> [w433]
                  tunnel: w146 -> [w403]
                  stop <- w453 stop-if-true
                  w416 = T1."Idle"
                  # "Ephys Trigger"
                  # "Pool 100 cycles"
                  # "ADD TRIAL #, Start and end of trial"
                  n234 = node-c288() -> (→"Actual cycle period (uS)":i64)  [unwired: 1 in, 1 out]
                  n235 = local read "Lick reward"() -> (w471:bool)
                  n236 = local read "Reward period (uS)"() -> (w432:u32)
                  n237 = call-poly <vilib>:"DAQmx Read.vi"("task/channels in"=w452, "timeout"=0.1, "error in"=w451) -> ("task out"=w445:refnum<k21>, "data"=w448:dbl[], "error out"=w446:errorcluster)  [unwired: 10 in]
                  n238 = local read "Reward start delay (uS)"() -> (w428:u32)
                  n239 = call "Tick Count"() -> ("Tick Count(uSec)"=w479:u32)
                  n240 = Index Array(array=w448, index #1=0 ("index"), index #2=1 ("index"), index #3=2 ("index"), index #4=3 ("index"), index #5=4 ("index")) -> (element #1=w439:dbl, element #2=w447:dbl, element #3=w406:dbl, element #4=w402:dbl, element #5=w409:dbl)
                  n241 = feedback #1(FALSE) -> (w474:bool)
                  n242 = feedback-in #1(w471) -> ()
                  n243 = feedback #2(w479) -> (w480:u32)
                  n244 = feedback-in #2(w479) -> ()
                  n245 = local read "Trial timeout (uS)"() -> (w426:u32)
                  n246 = Greater?(x=w471, y=w474) -> (0:w472:bool)
                  n247 = Subtract(x=w479, y=w480) -> (x-y=w478:u32)
                  n248 = call "vs digital filter3.vi"("filter period(uSec)"=w404, "vs threshold"=w405, "input"=w406) -> ("output"=w399:bool)  [unwired: 3 in]
                  n249 = To Unsigned Quad Integer(1:w478) -> (0:w477:u64)
                  n250 = Greater?(x=w447, y=w438) -> (0:w398:bool)
                  n251 = feedback #3(u64 0) -> (w476:u64)
                  n252 = Add(x=w477, y=w476) -> (x+y=w430:u64)
                  n253 = Divide(x=w430, y=u64 1000) -> (x/y=w469:dbl)
                  n254 = feedback-in #3(w430) -> ()
                  n255 = call "vs digital filter.vi"("filter period(uSec)"=w404, "vs threshold"=w405, "input"=w439) -> ("output"=w401:bool)  [unwired: 3 in]
                  n256 = feedback #4(w416) -> (w481:T1)
                  n257 = Select(t=T1."Lick reward", s=w472, f=w481) -> (s? t:f=w412:T1)
                  n258 = feedback #5(w416) -> (w417:T1)
                  n259 = local read "ABORT"() -> (w453:bool)
                  n260 = case shown="\"After VS\"" w412 {
                    selector: w412 -> [w490 w496 w510 w527 w534 w555 _ w573 w600 w618 w636 w645 w651 w675]
                    tunnel: w436 -> [w491 w505 w515 w531 w552 w561 w570 w586 w604 w620 w640 w647 w663 w678]
                    tunnel: w435 -> [w487 w504 w514 w530 w550 w560 w569 w584 w603 w619 w639 w646 w662 w680]
                    tunnel: w398 -> [_ _ _ _ w538 _ _ _ _ _ _ _ _ w674]
                    tunnel: w434 -> [w486 w503 w513 w529 w542 w559 w566 w583 w590 w616 w634 w644 w657 w673]
                    tunnel: w433 -> [w485 w502 w511 w524 w548 w558 w565 w582 w596 w615 w633 w643 w660 w672]
                    tunnel: w432 -> [_ _ _ _ w546 _ _ _ _ _ _ _ _ _]
                    tunnel: w431 -> [_ _ _ _ _ _ _ w581 _ _ _ _ _ w671]
                    tunnel: w430 -> [_ _ _ w521 w541 _ _ w576 w593 w609 w625 _ w654 w667]
                    tunnel: w429 -> [w484 w501 w512 w528 w547 w557 w564 w578 w595 w614 w631 w642 w659 w668]
                    tunnel: w428 -> [_ _ _ w522 _ _ _ _ _ _ _ _ _ _]
                    tunnel: w427 -> [_ _ _ _ _ _ _ _ _ _ _ _ _ _]
                    tunnel: w426 -> [_ _ _ _ _ _ _ _ w599 _ _ _ w655 _]
                    tunnel: w425 -> [_ _ _ _ _ _ _ _ _ w611 _ _ _ _]
                    tunnel: w424 -> [_ _ _ _ _ _ _ _ _ _ w629 _ _ _]
                    tunnel: [w491 w505 w515 w531 w552 w561 w570 w585 w604 w620 w640 w647 w663 w679] -> w423
                    tunnel: [w487 w504 w514 w530 w550 w560 w568 w584 w603 w619 w639 w646 w662 w680] -> w422
                    tunnel: [w488 w499 w507 w516 w551 w555 T1."Idle" w575 w602 w605 w638 w645 w653 w676] -> w413
                    tunnel: [FALSE FALSE FALSE FALSE FALSE FALSE FALSE TRUE FALSE FALSE FALSE FALSE FALSE w674] -> w421
                    tunnel: [w486 w503 w513 w529 w540 w559 w566 w583 w590 w616 w634 w644 w650 w673] -> w420
                    tunnel: [w484 w501 w512 w528 w547 w557 w564 w577 w594 w606 w627 w642 w659 w665] -> w419
                    tunnel: [w485 w502 w511 w519 w548 w558 w565 w582 w596 w615 w633 w643 w660 w672] -> w418
                    tunnel: w417 -> [_ _ _ w526 w545 _ _ w588 w601 w617 w635 _ w661 w677]
                    tunnel: w401 -> [_ w498 w506 _ _ _ _ _ _ _ w626 _ _ _]
                    frame "Idle", Default {
                      n261 = local read "Start one trial"() -> (w489:bool)
                      n262 = case shown="True" w489 {
                        tunnel: w490 -> [w492 _]
                        tunnel: [w492 w493] -> w488
                        frame False {
                        }
                        frame True {
                          n263 = stacked-sequence {
                            tunnel: [T1."Before VS" _] -> w493
                            frame #0 {
                            }
                            frame #1 {
                              w495 = FALSE
                              n264 = local write "Start one trial"(w495) -> ()
                              n265 = local write "Trial Done"(w495) -> ()
                            }
                          }
                        }
                      }
                    }
                    frame "Before VS" {
                      n266 = Select(t=T1."VS", s=w498, f=w496) -> (s? t:f=w499:T1)
                    }
                    frame "VS" {
                      n267 = Select(t=w510, s=w506, f=T1."After VS") -> (s? t:f=w507:T1)
                    }
                    frame "VS2" {
                      n268 = Equal?(x=w527, y=w526) -> (x = y?=w525:bool)
                      n269 = Add(x=w521, y=w522) -> (x+y=w523:u64)
                      n270 = Select(t=w524, s=w525, f=w523) -> (s? t:f=w519:u64)
                      n271 = Greater?(x=w519, y=w521) -> (0:w520:bool)
                      n272 = Select(t=w527, s=w520, f=T1."After VS") -> (s? t:f=w516:T1)
                    }
                    frame "After VS" {
                      n273 = Equal?(x=w534, y=w545) -> (x = y?=w543:bool)
                      n274 = Add(x=w546, y=w541) -> (x+y=w544:u64)
                      n275 = Select(t=w542, s=w543, f=w544) -> (s? t:f=w540:u64)
                      n276 = Greater?(x=w540, y=w541) -> (0:w539:bool)
                      n277 = Select(t=T1."Reward", s=w538, f=w534) -> (s? t:f=w535:T1)
                      n278 = Select(t=w535, s=w539, f=T1."Cycle End") -> (s? t:f=w549:T1)
                      n279 = case shown="True" "Automatic reward" {
                        tunnel: [w553 T1."Reward"] -> w551
                        tunnel: w549 -> [w553 _]
                        frame False {
                        }
                        frame True {
                        }
                      }
                    }
                    frame "Wait for lever press" {
                    }
                    frame "Cycle End" {
                      n280 = Increment(x=w569) -> (x+1=w568:i32)
                      n281 = local write "Trial Done"(TRUE) -> ()
                    }
                    frame "Reward" {
                      n282 = Add(x=w581, y=w576) -> (x+y=w580:u64)
                      n283 = Increment(x=w586) -> (x+1=w587:i32)
                      n284 = Equal?(x=w573, y=w588) -> (x = y?=w579:bool)
                      n285 = Select(t=w578, s=w579, f=w580) -> (s? t:f=w577:u64)
                      n286 = Select(t=w586, s=w579, f=w587) -> (s? t:f=w585:i32)
                      "# of rewards" <- w585
                      n287 = Greater?(x=w577, y=w576) -> (0:w574:bool)
                      n288 = Select(t=w573, s=w574, f=T1."Cycle End") -> (s? t:f=w575:T1)
                    }
                    frame "Reward Refractory" {
                      n289 = Equal?(x=w600, y=w601) -> (x = y?=w597:bool)
                      n290 = Add(x=w593, y=w599) -> (x+y=w598:u64)
                      n291 = Select(t=w595, s=w597, f=w598) -> (s? t:f=w594:u64)
                      n292 = Greater?(x=w594, y=w593) -> (0:w592:bool)
                      n293 = Select(t=w600, s=w592, f=T1."Cycle End") -> (s? t:f=w602:T1)
                    }
                    frame "Punish" {
                      n294 = Equal?(x=w618, y=w617) -> (x = y?=w613:bool)
                      n295 = Add(x=w609, y=w611) -> (x+y=w612:u64)
                      n296 = Select(t=w614, s=w613, f=w612) -> (s? t:f=w606:u64)
                      n297 = Greater?(x=w606, y=w609) -> (0:w610:bool)
                      n298 = Select(t=w618, s=w610, f=T1."Punish Refractory") -> (s? t:f=w605:T1)
                    }
                    frame "Punish Refractory" {
                      n299 = Equal?(x=w636, y=w635) -> (x = y?=w632:bool)
                      n300 = Add(x=w625, y=w629) -> (x+y=w630:u64)
                      n301 = Select(t=w631, s=w632, f=w630) -> (s? t:f=w624:u64)
                      n302 = Greater?(x=w624, y=w625) -> (0:w628:bool)
                      n303 = Select(t=w636, s=w628, f=T1."Before VS") -> (s? t:f=w637:T1)
                      n304 = Select(t=w625, s=w626, f=w624) -> (s? t:f=w627:u64)
                      n305 = Select(t=T1."VS2", s=w626, f=w637) -> (s? t:f=w638:T1)
                    }
                    frame "Exit" {
                    }
                    frame "Timeout" {
                      n306 = Equal?(x=w651, y=w661) -> (x = y?=w658:bool)
                      n307 = Add(x=w654, y=w655) -> (x+y=w656:u64)
                      n308 = Select(t=w657, s=w658, f=w656) -> (s? t:f=w650:u64)
                      n309 = Greater?(x=w650, y=w654) -> (0:w652:bool)
                      n310 = Select(t=w651, s=w652, f=T1."Cycle End") -> (s? t:f=w653:T1)
                    }
                    frame "Lick reward" {
                      n311 = Equal?(x=w675, y=w677) -> (x = y?=w670:bool)
                      n312 = Add(x=w671, y=w667) -> (x+y=w669:u64)
                      n313 = Select(t=w668, s=w670, f=w669) -> (s? t:f=w665:u64)
                      n314 = Greater?(x=w665, y=w667) -> (0:w666:bool)
                      n315 = case shown="True" w674 {
                        tunnel: [w681 w683] -> w679
                        tunnel: w678 -> [w681 w682]
                        frame False {
                        }
                        frame True {
                          n316 = Increment(x=w682) -> (x+1=w683:i32)
                        }
                      }
                      n317 = Select(t=w675, s=w666, f=T1."Reward Refractory") -> (s? t:f=w676:T1)
                    }
                  }
                  n318 = Build Array(w469, w435, w412, w402) -> (w395:dbl[])
                  n319 = To Single Precision Float(number=w395) -> (single precision float=w396:sgl[])
                  n320 = local read "Manually give water"() -> (w470:bool)
                  n321 = shared-variable "My Computer\\Network variables.lvlib\\stop - network"() -> (w482:bool)  [unwired: 1 in, 1 out]
                  n322 = Select(t=T1."Exit", s=w482, f=w413) -> (s? t:f=w437:T1)
                  n323 = feedback-in #4(w437) -> ()
                  n324 = feedback-in #5(w437) -> ()
                  n325 = Or(x=w470, y=w421) -> (x .or. y?=w397:bool)
                  n326 = Build Array(w399, w398, w397) -> (w456:bool[])
                  n327 = Boolean Array To Number(Boolean array=w456) -> (number=w393:u32)
                  n328 = To Single Precision Float(number=w393) -> (single precision float=w394:sgl)
                  n329 = Build Array (concatenate)(w396, w394) -> (w455:sgl[])
                  n330 = Build Array (concatenate)(w467, w455) -> (w463:sgl[])
                  n331 = Array Size(array=w463) -> (size(s)=w458:i32)
                  n332 = Equal?(x=w458, y=w403) -> (x = y?=w457:bool)
                  n333 = case shown="True" w457 {
                    tunnel: w466 -> [_ w696]
                    tunnel: [w686 w695] -> w465
                    tunnel: w464 -> [w686 w693]
                    tunnel: w463 -> [w685 w690]
                    tunnel: [w685 sgl[] [] ("array type (2D Dbl)")] -> w462
                    tunnel: w461 -> [_ w689]
                    tunnel: w460 -> [w684 w688]
                    tunnel: [w684 w687] -> w459
                    frame False {
                    }
                    frame True {
                      n334 = RT FIFO Write(0:w696, 1:w690, 2:10 ("timeout in ms (0)"), 3:w693) -> (11:w695:errorcluster)  [unwired: 1 in, 3 out]
                      n335 = RT FIFO Write(0:w689, 1:w690, 2:10 ("timeout in ms (0)"), 3:w688) -> (11:w687:errorcluster)  [unwired: 1 in, 3 out]
                    }
                  }
                  n336 = call "vs digital filter2.vi"("filter period(uSec)"=w404, "vs threshold"=w405, "input"=w409) -> ("output"=w400:bool)  [unwired: 3 in]
                  n337 = Build Array(w397, w400, w399) -> (w444:bool[])
                  n338 = node-c288() -> ()  [unwired: 3 in, 1 out]
                  n339 = call-poly <vilib>:"DAQmx Write.vi"("task/channels in"=w443, "data"=w444, "error in"=w442) -> ("task out"=w440:refnum<k21>, "error out"=w441:errorcluster)  [unwired: 10 in, 1 out]
                }
                n340 = node-c288(w206) -> (w199:errorcluster)
                n341 = call <vilib>:"DAQmx Stop Task.vi"("task/channels in"=w163, "error in"=w164) -> ("error out"=w162:errorcluster)  [unwired: 12 in, 1 out]
                n342 = Merge Errors(w193, w196, w188, w187) -> (w195:errorcluster)
                n343 = Build Array(w155, w155, w155) -> (w157:bool[])
                n344 = call-poly <vilib>:"DAQmx Write.vi"("task/channels in"=w161, "data"=w157, "error in"=w160) -> ("task out"=w159:refnum<k21>, "error out"=w158:errorcluster)  [unwired: 10 in, 1 out]
                n345 = call <vilib>:"DAQmx Stop Task.vi"("task/channels in"=w159, "error in"=w158) -> ("error out"=w177:errorcluster)  [unwired: 12 in, 1 out]
                n346 = Merge Errors(w162, w177) -> (w197:errorcluster)
                n347 = stacked-sequence {
                  tunnel: w214 -> [w712]
                  tunnel: w215 -> [w711]
                  tunnel: w201 -> [w709]
                  tunnel: w200 -> [w708]
                  tunnel: w199 -> [w707]
                  tunnel: w197 -> [w706]
                  tunnel: w195 -> [w705]
                  frame #0 {
                    n348 = Merge Errors(w707, w708, w712, w711, w709, w706, w705) -> (w710:errorcluster)
                    "error out" <- w710
                    n349 = call <vilib>:"Simple Error Handler.vi"("error in (no error)"=w710) -> ()  [unwired: 4 in, 5 out]
                  }
                }
              }
            }
          }
          frame #2 {
            n350 = Wait (ms)(milliseconds to wait=u32 50) -> ()  [unwired: 1 out]
          }
        }
      }
      n351 = UDP Close(connection ID=w2, 8:w3) -> (error out=w1:errorcluster)  [unwired: 1 out]
      n352 = call <vilib>:"Simple Error Handler.vi"("error in (no error)"=w1) -> ()  [unwired: 4 in, 5 out]
    }
    frame #1 {
      w947 = FALSE
      n353 = local write "Busy"(w947) -> ()
      n354 = local write "ABORT"(w947) -> ()
      n355 = local write "Initial data received"(w947) -> ()
      n356 = local write "Stop state"(w947) -> ()
    }
  }
